vi "get id.vi"(8 "error in (no error)":errorcluster, 11 "Variant (Cluster) in":variant) -> (0 "error out":errorcluster, 1 "found?":bool, 2 "id":variant, 3 "Variant (Cluster) out":variant)   [LabVIEW 2017, in "JSONRPC Server.lvclass"]
uses:
  JSONRPC Server.lvclass
  <vilib>/National Instruments/Variant Data Manipulation/Variant Data Manipulation.lvlib
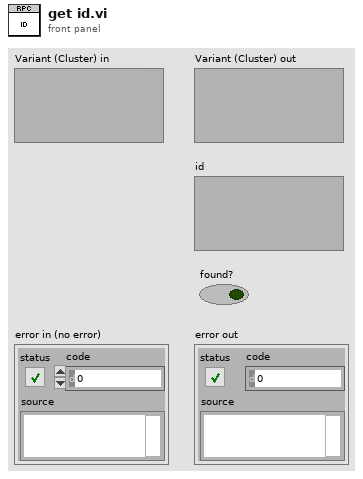
[diagram p1: front panel]
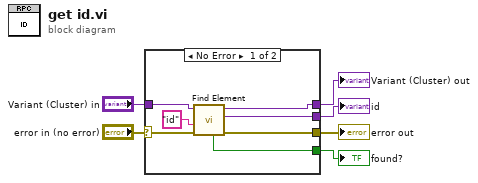
[diagram p0: block diagram]
diagram:
  n1 = case shown="No Error" "error in (no error)" {
    selector: "error in (no error)" -> [w12 w14]
    tunnel: [w13 w14] -> w6
    tunnel: [w11 w15] -> w4
    tunnel: [w10 _] -> w3
    tunnel: "Variant (Cluster) in" -> [w9 w15]
    tunnel: [w8 _] -> w1
    frame No Error {
      n2 = call <vilib>:"Find Element.vi"("error in (no error)"=w12, "Name"="id", "Variant (Cluster) in"=w9) -> ("error out"=w13:errorcluster, "element"=w8:variant, "Variant (Cluster) out"=w11:variant, "found?"=w10:bool)  [unwired: 4 in, 1 out]
    }
    frame Error {
    }
  }
  "error out" <- w6
  "Variant (Cluster) out" <- w4
  "found?" <- w3
  "id" <- w1
